vi "23384_Davis_Poku_Amankwa_Amankwa.DavisPoku.MNE1201.8.4_348265_949570043.vi"() -> ()   [LabVIEW 2018]
panel:
  in  "stop":bool
  out "Waveform Chart 2":dbl(graph)
  out "Waveform Chart 1":dbl(graph)
  # "4a. Only one waveform chart was executing, and this is because since labview operates by default in sequential processes, the code was waiting for the first while loop to finish executing before it carries on to the second"
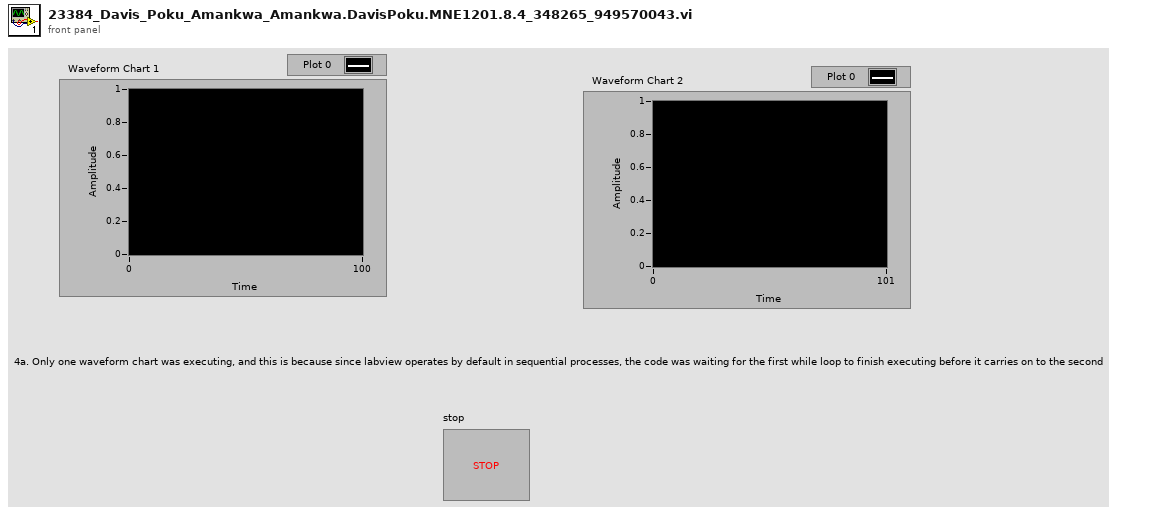
[diagram p1: front panel]
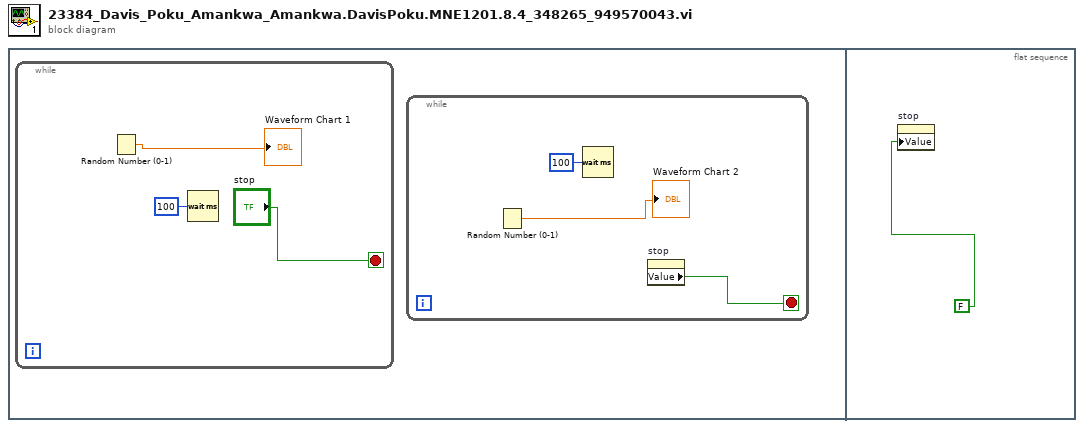
[diagram p0: block diagram]
diagram:
  n1 = flat-sequence {
    frame #0 {
      n2 = while {
        stop <- "stop" stop-if-true
        n3 = Random Number (0-1)() -> (number: 0 to 1=→"Waveform Chart 1":dbl)
        n4 = Wait (ms)(milliseconds to wait=u32 100) -> ()  [unwired: 1 out]
      }
      n5 = while {
        stop <- w1 stop-if-true
        n6 = Random Number (0-1)() -> (number: 0 to 1=→"Waveform Chart 2":dbl)
        n7 = Wait (ms)(milliseconds to wait=u32 100) -> ()  [unwired: 1 out]
        n8 = property on="stop" class="Bool (strict)"() -> ("Value"=w1:bool)  [unwired: 2 in, 2 out]
      }
    }
    frame #1 {
      n9 = property on="stop" class="Bool (strict)"("Value"=FALSE) -> ()  [unwired: 2 in, 2 out]
    }
  }
